vi "Lab Panel V5.29.vi"() -> ()   [LabVIEW 2013] (continued)
                        n3233 = local read "LAB03 TEMP"() -> (w5903:T12)
                        n3234 = call "sub vi - temperature delay v4.vi"("2-run"=w5884, "1-run"=w5885, "temp values IN"=w5902, "temp signals"=w5903) -> ("T2-N"=w5897:dbl, "T2-L"=w5898:dbl, "T1-N"=w5899:dbl, "T1-L"=w5900:dbl, "temp values OUT"=w5901:T44)  [unwired: 3 in]
                        n3235 = Unbundle By Name(w5912) -> ("1 (TL) cal"=w5907:dbl, "1 (TN) cal"=w5906:dbl, "2 (TL) cal"=w5905:dbl, "2 (TN) cal"=w5904:dbl)  [unwired: 6 out]
                        n3236 = local write "TEMP LA03"(w5901) -> ()
                        n3237 = Multiply(x=w5900, y=w5907) -> (x*y=w5893:dbl)
                        n3238 = Multiply(x=w5899, y=w5906) -> (x*y=w5892:dbl)
                        n3239 = Multiply(x=w5898, y=w5905) -> (x*y=w5889:dbl)
                        n3240 = Multiply(x=w5897, y=w5904) -> (x*y=w5888:dbl)
                        n3241 = case shown="True" w5884 {
                          tunnel: w5889 -> [w5914 w5919]
                          tunnel: w5894 -> [_ w5917]
                          tunnel: [w5914 w5918] -> w5887
                          tunnel: w5888 -> [w5913 w5916]
                          tunnel: [w5913 w5915] -> w5886
                          frame False {
                          }
                          frame True {
                            n3242 = Multiply(x=w5917, y=w5916) -> (x*y=w5915:dbl)
                            n3243 = Multiply(x=w5917, y=w5919) -> (x*y=w5918:dbl)
                          }
                        }
                        n3244 = case shown="True" w5885 {
                          tunnel: w5893 -> [w5921 w5926]
                          tunnel: w5894 -> [_ w5924]
                          tunnel: [w5921 w5925] -> w5891
                          tunnel: w5892 -> [w5920 w5923]
                          tunnel: [w5920 w5922] -> w5890
                          frame False {
                          }
                          frame True {
                            n3245 = Multiply(x=w5924, y=w5923) -> (x*y=w5922:dbl)
                            n3246 = Multiply(x=w5924, y=w5926) -> (x*y=w5925:dbl)
                          }
                        }
                        n3247 = local read "SIG LAB03-2"() -> (w5909:T2)
                        n3248 = local read "SIG LAB03-1"() -> (w5911:T2)
                        n3249 = Bundle By Name(cluster=w5911, "Tmp Live"=w5891, "Tmp Neut"=w5890) -> (w5910:T2)
                        n3250 = Bundle By Name(cluster=w5909, "Tmp Live"=w5887, "Tmp Neut"=w5886) -> (w5908:T2)
                        n3251 = local write "SIG LAB03-1"(w5910) -> ()
                        n3252 = local write "SIG LAB03-2"(w5908) -> ()
                      }
                      frame #4 {
                        n3253 = case shown="False" w5941 {
                          tunnel: [w5972 w5973] -> w5957
                          tunnel: w5940 -> [_ w5973]
                          frame False {
                            n3254 = local read "CAL LAB04"() -> (w5972:T14)
                          }
                          frame True {
                          }
                        }
                        n3255 = local read "LAB04 TEMP"() -> (w5947:T12)
                        n3256 = local read "TEMP LA04"() -> (w5948:T9)
                        n3257 = call "sub vi - temperature delay v4.vi"("2-run"=w5929, "1-run"=w5930, "temp values IN"=w5948, "temp signals"=w5947) -> ("T2-N"=w5942:dbl, "T2-L"=w5943:dbl, "T1-N"=w5944:dbl, "T1-L"=w5945:dbl, "temp values OUT"=w5946:T44)  [unwired: 3 in]
                        n3258 = Unbundle By Name(w5957) -> ("1 (TL) cal"=w5952:dbl, "1 (TN) cal"=w5951:dbl, "2 (TL) cal"=w5950:dbl, "2 (TN) cal"=w5949:dbl)  [unwired: 6 out]
                        n3259 = local write "TEMP LA04"(w5946) -> ()
                        n3260 = Multiply(x=w5945, y=w5952) -> (x*y=w5938:dbl)
                        n3261 = Multiply(x=w5944, y=w5951) -> (x*y=w5937:dbl)
                        n3262 = Multiply(x=w5943, y=w5950) -> (x*y=w5934:dbl)
                        n3263 = Multiply(x=w5942, y=w5949) -> (x*y=w5933:dbl)
                        n3264 = case shown="True" w5929 {
                          tunnel: w5934 -> [w5959 w5964]
                          tunnel: w5939 -> [_ w5962]
                          tunnel: [w5959 w5963] -> w5932
                          tunnel: w5933 -> [w5958 w5961]
                          tunnel: [w5958 w5960] -> w5931
                          frame False {
                          }
                          frame True {
                            n3265 = Multiply(x=w5962, y=w5961) -> (x*y=w5960:dbl)
                            n3266 = Multiply(x=w5962, y=w5964) -> (x*y=w5963:dbl)
                          }
                        }
                        n3267 = case shown="True" w5930 {
                          tunnel: w5938 -> [w5966 w5971]
                          tunnel: w5939 -> [_ w5969]
                          tunnel: [w5966 w5970] -> w5936
                          tunnel: w5937 -> [w5965 w5968]
                          tunnel: [w5965 w5967] -> w5935
                          frame False {
                          }
                          frame True {
                            n3268 = Multiply(x=w5969, y=w5968) -> (x*y=w5967:dbl)
                            n3269 = Multiply(x=w5969, y=w5971) -> (x*y=w5970:dbl)
                          }
                        }
                        n3270 = local read "SIG LAB04-2"() -> (w5954:T2)
                        n3271 = local read "SIG LAB04-1"() -> (w5956:T2)
                        n3272 = Bundle By Name(cluster=w5956, "Tmp Live"=w5936, "Tmp Neut"=w5935) -> (w5955:T2)
                        n3273 = Bundle By Name(cluster=w5954, "Tmp Live"=w5932, "Tmp Neut"=w5931) -> (w5953:T2)
                        n3274 = local write "SIG LAB04-1"(w5955) -> ()
                        n3275 = local write "SIG LAB04-2"(w5953) -> ()
                      }
                      frame #5 {
                        n3276 = case shown="False" w5986 {
                          tunnel: [w6017 w6018] -> w6002
                          tunnel: w5985 -> [_ w6018]
                          frame False {
                            n3277 = local read "CAL LAB05"() -> (w6017:T14)
                          }
                          frame True {
                          }
                        }
                        n3278 = local read "LAB05 TEMP"() -> (w5992:T12)
                        n3279 = local read "TEMP LA05"() -> (w5993:T9)
                        n3280 = call "sub vi - temperature delay v4.vi"("2-run"=w5974, "1-run"=w5975, "temp values IN"=w5993, "temp signals"=w5992) -> ("T2-N"=w5988:dbl, "T2-L"=w5989:dbl, "T1-N"=w5990:dbl, "T1-L"=w5991:dbl, "temp values OUT"=w5987:T44)  [unwired: 3 in]
                        n3281 = local write "TEMP LA05"(w5987) -> ()
                        n3282 = Unbundle By Name(w6002) -> ("1 (TL) cal"=w5994:dbl, "1 (TN) cal"=w5997:dbl, "2 (TL) cal"=w5996:dbl, "2 (TN) cal"=w5995:dbl)  [unwired: 6 out]
                        n3283 = Multiply(x=w5991, y=w5994) -> (x*y=w5983:dbl)
                        n3284 = Multiply(x=w5990, y=w5997) -> (x*y=w5982:dbl)
                        n3285 = Multiply(x=w5989, y=w5996) -> (x*y=w5979:dbl)
                        n3286 = Multiply(x=w5988, y=w5995) -> (x*y=w5978:dbl)
                        n3287 = case shown="True" w5974 {
                          tunnel: w5979 -> [w6004 w6009]
                          tunnel: w5984 -> [_ w6007]
                          tunnel: [w6004 w6008] -> w5977
                          tunnel: w5978 -> [w6003 w6006]
                          tunnel: [w6003 w6005] -> w5976
                          frame False {
                          }
                          frame True {
                            n3288 = Multiply(x=w6007, y=w6006) -> (x*y=w6005:dbl)
                            n3289 = Multiply(x=w6007, y=w6009) -> (x*y=w6008:dbl)
                          }
                        }
                        n3290 = case shown="True" w5975 {
                          tunnel: w5983 -> [w6011 w6016]
                          tunnel: w5984 -> [_ w6014]
                          tunnel: [w6011 w6015] -> w5981
                          tunnel: w5982 -> [w6010 w6013]
                          tunnel: [w6010 w6012] -> w5980
                          frame False {
                          }
                          frame True {
                            n3291 = Multiply(x=w6014, y=w6013) -> (x*y=w6012:dbl)
                            n3292 = Multiply(x=w6014, y=w6016) -> (x*y=w6015:dbl)
                          }
                        }
                        n3293 = local read "SIG LAB05-1"() -> (w6001:T2)
                        n3294 = Bundle By Name(cluster=w6001, "Tmp Live"=w5981, "Tmp Neut"=w5980) -> (w6000:T2)
                        n3295 = local read "SIG LAB05-2"() -> (w5999:T2)
                        n3296 = Bundle By Name(cluster=w5999, "Tmp Live"=w5977, "Tmp Neut"=w5976) -> (w5998:T2)
                        n3297 = local write "SIG LAB05-1"(w6000) -> ()
                        n3298 = local write "SIG LAB05-2"(w5998) -> ()
                      }
                      frame #6 {
                        w6119 = 150.0
                        # "check for thermocouple error, output >150 deg??"
                        n3299 = local read "SIG LAB01-2"() -> (w6128:T2)
                        n3300 = local read "SIG LAB04-1"() -> (w6122:T2)
                        n3301 = local read "SIG LAB04-2"() -> (w6123:T2)
                        n3302 = local read "SIG LAB01-1"() -> (w6129:T2)
                        n3303 = Unbundle(w6123) -> ("Tmp Live"=w6033:dbl, "Tmp Neut"=w6032:dbl)  [unwired: 3 out]
                        n3304 = Unbundle(w6128) -> ("Tmp Live"=w6054:dbl, "Tmp Neut"=w6052:dbl)  [unwired: 3 out]
                        n3305 = Unbundle(w6122) -> ("Tmp Live"=w6034:dbl, "Tmp Neut"=w6027:dbl)  [unwired: 3 out]
                        n3306 = Unbundle(w6129) -> ("Tmp Live"=w6057:dbl, "Tmp Neut"=w6055:dbl)  [unwired: 3 out]
                        n3307 = Absolute Value(x=w6034) -> (abs(x)=w6028:dbl)
                        n3308 = Absolute Value(x=w6027) -> (abs(x)=w6029:dbl)
                        n3309 = Absolute Value(x=w6033) -> (abs(x)=w6031:dbl)
                        n3310 = Absolute Value(x=w6032) -> (abs(x)=w6030:dbl)
                        n3311 = Absolute Value(x=w6054) -> (abs(x)=w6053:dbl)
                        n3312 = Absolute Value(x=w6052) -> (abs(x)=w6051:dbl)
                        n3313 = Absolute Value(x=w6055) -> (abs(x)=w6056:dbl)
                        n3314 = Absolute Value(x=w6057) -> (abs(x)=w6058:dbl)
                        n3315 = Greater?(x=w6030, y=w6119) -> (0:w6095:bool)
                        "LA04-2 (TN)" <- w6095
                        n3316 = Greater?(x=w6051, y=w6119) -> (0:w6107:bool)
                        "LA01-2 (TN)" <- w6107
                        n3317 = Greater?(x=w6031, y=w6119) -> (0:w6096:bool)
                        "LA04-2 (TL)" <- w6096
                        n3318 = Greater?(x=w6053, y=w6119) -> (0:w6108:bool)
                        "LA01-2 (TL)" <- w6108
                        n3319 = Greater?(x=w6029, y=w6119) -> (0:w6097:bool)
                        "LA04-1 (TN)" <- w6097
                        n3320 = Greater?(x=w6056, y=w6119) -> (0:w6118:bool)
                        "LA01-1 (TN)" <- w6118
                        n3321 = Greater?(x=w6028, y=w6119) -> (0:w6098:bool)
                        "LA04-1 (TL)" <- w6098
                        n3322 = Greater?(x=w6058, y=w6119) -> (0:w6117:bool)
                        "LA01-1 (TL)" <- w6117
                        n3323 = Or(x=w6118, y=w6117) -> (x .or. y?=w6116:bool)
                        n3324 = Or(x=w6095, y=w6096) -> (x .or. y?=w6106:bool)
                        n3325 = Or(x=w6108, y=w6107) -> (x .or. y?=w6112:bool)
                        n3326 = Or(x=w6097, y=w6098) -> (x .or. y?=w6102:bool)
                        n3327 = Select(t=u32 16711680, s=w6116, f=u32 13816530) -> (s? t:f=w6113:u32)
                        n3328 = Select(t=u32 16711680, s=w6106, f=u32 13816530) -> (s? t:f=w6103:u32)
                        n3329 = Select(t=u32 16711680, s=w6112, f=u32 13816530) -> (s? t:f=w6109:u32)
                        n3330 = Select(t=u32 16711680, s=w6102, f=u32 13816530) -> (s? t:f=w6099:u32)
                        n3331 = property on="SIG LAB01-1" class="Clust (strict)"("Color"=w6113) -> ()  [unwired: 2 in, 2 out]
                        n3332 = property on="SIG LAB01-2" class="Clust (strict)"("Color"=w6109) -> ()  [unwired: 2 in, 2 out]
                        n3333 = property on="SIG LAB04-2" class="Clust (strict)"("Color"=w6103) -> ()  [unwired: 2 in, 2 out]
                        n3334 = property on="SIG LAB04-1" class="Clust (strict)"("Color"=w6099) -> ()  [unwired: 2 in, 2 out]
                        n3335 = local read "SIG LAB02-1"() -> (w6126:T2)
                        n3336 = local read "SIG LAB02-2"() -> (w6127:T2)
                        n3337 = local read "SIG LAB05-2"() -> (w6120:T2)
                        n3338 = local read "SIG LAB05-1"() -> (w6121:T2)
                        n3339 = Unbundle(w6127) -> ("Tmp Live"=w6046:dbl, "Tmp Neut"=w6044:dbl)  [unwired: 3 out]
                        n3340 = Unbundle(w6126) -> ("Tmp Live"=w6050:dbl, "Tmp Neut"=w6049:dbl)  [unwired: 3 out]
                        n3341 = Unbundle(w6120) -> ("Tmp Live"=w6022:dbl, "Tmp Neut"=w6020:dbl)  [unwired: 3 out]
                        n3342 = Unbundle(w6121) -> ("Tmp Live"=w6026:dbl, "Tmp Neut"=w6024:dbl)  [unwired: 3 out]
                        n3343 = Absolute Value(x=w6046) -> (abs(x)=w6045:dbl)
                        n3344 = Absolute Value(x=w6044) -> (abs(x)=w6043:dbl)
                        n3345 = Absolute Value(x=w6049) -> (abs(x)=w6047:dbl)
                        n3346 = Absolute Value(x=w6050) -> (abs(x)=w6048:dbl)
                        n3347 = Absolute Value(x=w6022) -> (abs(x)=w6021:dbl)
                        n3348 = Absolute Value(x=w6020) -> (abs(x)=w6019:dbl)
                        n3349 = Absolute Value(x=w6026) -> (abs(x)=w6025:dbl)
                        n3350 = Absolute Value(x=w6024) -> (abs(x)=w6023:dbl)
                        n3351 = Greater?(x=w6043, y=w6119) -> (0:w6071:bool)
                        "LA02-2 (TN)" <- w6071
                        n3352 = Greater?(x=w6045, y=w6119) -> (0:w6072:bool)
                        "LA02-2 (TL)" <- w6072
                        n3353 = Greater?(x=w6047, y=w6119) -> (0:w6074:bool)
                        "LA02-1 (TN)" <- w6074
                        n3354 = Greater?(x=w6048, y=w6119) -> (0:w6073:bool)
                        "LA02-1 (TL)" <- w6073
                        n3355 = Greater?(x=w6019, y=w6119) -> (0:w6083:bool)
                        "LA05-2 (TN)" <- w6083
                        n3356 = Greater?(x=w6021, y=w6119) -> (0:w6084:bool)
                        "LA05-2 (TL)" <- w6084
                        n3357 = Greater?(x=w6023, y=w6119) -> (0:w6085:bool)
                        "LA05-1 (TN)" <- w6085
                        n3358 = Greater?(x=w6025, y=w6119) -> (0:w6086:bool)
                        "LA05-1 (TL)" <- w6086
                        n3359 = Or(x=w6074, y=w6073) -> (x .or. y?=w6082:bool)
                        n3360 = Or(x=w6072, y=w6071) -> (x .or. y?=w6078:bool)
                        n3361 = Or(x=w6086, y=w6085) -> (x .or. y?=w6094:bool)
                        n3362 = Or(x=w6084, y=w6083) -> (x .or. y?=w6090:bool)
                        n3363 = Select(t=u32 16711680, s=w6082, f=u32 13816530) -> (s? t:f=w6079:u32)
                        n3364 = Select(t=u32 16711680, s=w6078, f=u32 13816530) -> (s? t:f=w6075:u32)
                        n3365 = Select(t=u32 16711680, s=w6094, f=u32 13816530) -> (s? t:f=w6091:u32)
                        n3366 = Select(t=u32 16711680, s=w6090, f=u32 13816530) -> (s? t:f=w6087:u32)
                        n3367 = local read "SIG LAB03-1"() -> (w6124:T2)
                        n3368 = property on="SIG LAB02-1" class="Clust (strict)"("Color"=w6079) -> ()  [unwired: 2 in, 2 out]
                        n3369 = property on="SIG LAB02-2" class="Clust (strict)"("Color"=w6075) -> ()  [unwired: 2 in, 2 out]
                        n3370 = local read "SIG LAB03-2"() -> (w6125:T2)
                        n3371 = property on="SIG LAB05-1" class="Clust (strict)"("Color"=w6091) -> ()  [unwired: 2 in, 2 out]
                        n3372 = property on="SIG LAB05-2" class="Clust (strict)"("Color"=w6087) -> ()  [unwired: 2 in, 2 out]
                        n3373 = Unbundle(w6125) -> ("Tmp Live"=w6038:dbl, "Tmp Neut"=w6036:dbl)  [unwired: 3 out]
                        n3374 = Unbundle(w6124) -> ("Tmp Live"=w6042:dbl, "Tmp Neut"=w6040:dbl)  [unwired: 3 out]
                        n3375 = Absolute Value(x=w6038) -> (abs(x)=w6037:dbl)
                        n3376 = Absolute Value(x=w6036) -> (abs(x)=w6035:dbl)
                        n3377 = Absolute Value(x=w6042) -> (abs(x)=w6041:dbl)
                        n3378 = Absolute Value(x=w6040) -> (abs(x)=w6039:dbl)
                        n3379 = Greater?(x=w6035, y=w6119) -> (0:w6059:bool)
                        "LA03-2 (TN)" <- w6059
                        n3380 = Greater?(x=w6037, y=w6119) -> (0:w6060:bool)
                        "LA03-2 (TL)" <- w6060
                        n3381 = Greater?(x=w6039, y=w6119) -> (0:w6062:bool)
                        "LA03-1 (TN)" <- w6062
                        n3382 = Greater?(x=w6041, y=w6119) -> (0:w6061:bool)
                        "LA03-1 (TL)" <- w6061
                        n3383 = Or(x=w6062, y=w6061) -> (x .or. y?=w6070:bool)
                        n3384 = Or(x=w6060, y=w6059) -> (x .or. y?=w6066:bool)
                        n3385 = Select(t=u32 16711680, s=w6070, f=u32 13816530) -> (s? t:f=w6067:u32)
                        n3386 = Select(t=u32 16711680, s=w6066, f=u32 13816530) -> (s? t:f=w6063:u32)
                        n3387 = property on="SIG LAB03-1" class="Clust (strict)"("Color"=w6067) -> ()  [unwired: 2 in, 2 out]
                        n3388 = property on="SIG LAB03-2" class="Clust (strict)"("Color"=w6063) -> ()  [unwired: 2 in, 2 out]
                      }
                    }
                  }
                }
              }
            }
          }
          frame #22 {
            # "SAVE ON AMPS VALUES FOR REPORT FILE"
            # "write data to display panel"
            n3389 = global write "Global display 1.vi" "TEST 5-2"(w6165) -> ()
            n3390 = global write "Global display 1.vi" "TEST 4-2"(w6167) -> ()
            n3391 = global write "Global display 1.vi" "TEST 1-2"(w6173) -> ()
            n3392 = global write "Global display 1.vi" "TEST 3-1"(w6170) -> ()
            n3393 = global write "Global display 1.vi" "TEST 5-1"(w6166) -> ()
            n3394 = global write "Global display 1.vi" "TEST 1-1"(w6174) -> ()
            n3395 = global write "Global display 1.vi" "TEST 3-2"(w6169) -> ()
            n3396 = global write "Global display 1.vi" "TEST 4-1"(w6168) -> ()
            n3397 = global write "Global display 1.vi" "TEST 2-2"(w6171) -> ()
            n3398 = global write "Global display 1.vi" "TEST 2-1"(w6172) -> ()
            n3399 = global read "Global display 3.vi" "log 1-1"() -> (→"LOG LAB01-1":string)
            n3400 = global read "Global display 3.vi" "log 3-1"() -> (→"LOG LAB03-1":string)
            n3401 = global read "Global display 3.vi" "log 1-2"() -> (→"LOG LAB01-2":string)
            n3402 = property on="Tab Control 2" class="TabCtl (strict)"() -> ("Pages"=w6164:refnum<vi>[])  [unwired: 2 in, 2 out]
            n3403 = global read "Global display 3.vi" "log 2-1"() -> (→"LOG LAB02-1":string)
            n3404 = global read "Global display 3.vi" "log 2-2"() -> (→"LOG LAB02-2":string)
            n3405 = global read "Global display 3.vi" "log 4-2"() -> (→"LOG LAB04-2":string)
            n3406 = global read "Global display 3.vi" "log 5-2"() -> (→"LOG LAB05-2":string)
            n3407 = global read "Global display 3.vi" "log 5-1"() -> (→"LOG LAB05-1":string)
            n3408 = global read "Global display 3.vi" "log 4-1"() -> (→"LOG LAB04-1":string)
            n3409 = global read "Global display 3.vi" "log 3-2"() -> (→"LOG LAB03-2":string)
            n3410 = Index Array(array=w6164, index=8) -> (element=w6162:refnum<vi>)
            n3411 = property class="Page"(reference=w6162) -> ("PageVis"=w6161:bool)  [unwired: 1 in, 2 out]
            n3412 = global write "Global display 3.vi" "admin"(w6161) -> ()
            n3413 = local read "O/I  LAB05-2"() -> (w6215:bool)
            n3414 = local read "O/I  LAB05-1"() -> (w6216:bool)
            n3415 = local read "O/I  LAB03-2"() -> (w6219:bool)
            n3416 = local read "O/I  LAB04-2"() -> (w6217:bool)
            n3417 = local read "O/I  LAB04-1"() -> (w6218:bool)
            n3418 = local read "O/I  LAB03-1"() -> (w6220:bool)
            n3419 = local read "O/I  LAB01-2"() -> (w6223:bool)
            n3420 = local read "O/I  LAB01-1"() -> (w6224:bool)
            n3421 = local read "O/I  LAB02-1"() -> (w6222:bool)
            n3422 = local read "O/I  LAB02-2"() -> (w6221:bool)
            n3423 = global write "Global display 1.vi" "5-2 O/F"(w6215) -> ()
            n3424 = global write "Global display 1.vi" "5-1 O/F"(w6216) -> ()
            n3425 = global write "Global display 1.vi" "4-1 O/F"(w6218) -> ()
            n3426 = global write "Global display 1.vi" "4-2 O/F"(w6217) -> ()
            n3427 = global write "Global display 1.vi" "3-2 O/F"(w6219) -> ()
            n3428 = global write "Global display 1.vi" "3-1 O/F"(w6220) -> ()
            n3429 = global write "Global display 1.vi" "2-2 O/F"(w6221) -> ()
            n3430 = global write "Global display 1.vi" "2-1 O/F"(w6222) -> ()
            n3431 = global write "Global display 1.vi" "1-2 O/F"(w6223) -> ()
            n3432 = global write "Global display 1.vi" "1-1 O/F"(w6224) -> ()
            n3433 = local read "TEMP START LAB02-2"() -> (w6147:cluster{"TL":dbl, "TN":dbl})
            n3434 = local read "run lab05-2"() -> (w6205:bool)
            n3435 = local read "TEMP START LAB01-2"() -> (w6149:cluster{"TL":dbl, "TN":dbl})
            n3436 = local read "TEMP START LAB02-1"() -> (w6148:cluster{"TL":dbl, "TN":dbl})
            n3437 = local read "TEMP START LAB04-1"() -> (w6144:cluster{"TL":dbl, "TN":dbl})
            n3438 = local read "TEMP START LAB04-2"() -> (w6143:cluster{"TL":dbl, "TN":dbl})
            n3439 = local read "run lab04-1"() -> (w6208:bool)
            n3440 = local read "run lab04-2"() -> (w6207:bool)
            n3441 = local read "run lab05-1"() -> (w6206:bool)
            n3442 = local read "TEMP START LAB01-1"() -> (w6150:cluster{"TL":dbl, "TN":dbl})
            n3443 = local read "TEMP START LAB05-2"() -> (w6141:cluster{"TL":dbl, "TN":dbl})
            n3444 = local read "TEMP START LAB05-1"() -> (w6142:cluster{"TL":dbl, "TN":dbl})
            n3445 = local read "run lab03-2"() -> (w6209:bool)
            n3446 = local read "TEMP START LAB03-2"() -> (w6145:cluster{"TL":dbl, "TN":dbl})
            n3447 = local read "TEMP START LAB03-1"() -> (w6146:cluster{"TL":dbl, "TN":dbl})
            n3448 = local read "run lab02-1"() -> (w6212:bool)
            n3449 = local read "run lab03-1"() -> (w6210:bool)
            n3450 = local read "run lab01-2"() -> (w6213:bool)
            n3451 = local read "run lab02-2"() -> (w6211:bool)
            n3452 = local read "run lab01-1"() -> (w6214:bool)
            n3453 = global write "Global display 1.vi" "5-2 R/S"(w6205) -> ()
            n3454 = global write "Global display 1.vi" "5-1 R/S"(w6206) -> ()
            n3455 = global write "Global display 1.vi" "4-2 R/S"(w6207) -> ()
            n3456 = global write "Global display 1.vi" "4-1 R/S"(w6208) -> ()
            n3457 = global write "Global display 1.vi" "3-2 R/S"(w6209) -> ()
            n3458 = global write "Global display 1.vi" "1-2 R/S"(w6213) -> ()
            n3459 = global write "Global display 1.vi" "2-1 R/S"(w6212) -> ()
            n3460 = global write "Global display 1.vi" "3-1 R/S"(w6210) -> ()
            n3461 = global write "Global display 1.vi" "2-2 R/S"(w6211) -> ()
            n3462 = global write "Global display 1.vi" "1-1 R/S"(w6214) -> ()
            n3463 = global write "Global display 3.vi" "TEMP ST 05-2"(w6141) -> ()
            n3464 = global write "Global display 3.vi" "TEMP ST 05-1"(w6142) -> ()
            n3465 = global write "Global display 3.vi" "TEMP ST 03-2"(w6145) -> ()
            n3466 = global write "Global display 3.vi" "TEMP ST 04-2"(w6143) -> ()
            n3467 = global write "Global display 3.vi" "TEMP ST 01-1"(w6150) -> ()
            n3468 = global write "Global display 3.vi" "TEMP ST 01-2"(w6149) -> ()
            n3469 = global write "Global display 3.vi" "TEMP ST 04-1"(w6144) -> ()
            n3470 = global write "Global display 3.vi" "TEMP ST 02-1"(w6148) -> ()
            n3471 = global write "Global display 3.vi" "TEMP ST 02-2"(w6147) -> ()
            n3472 = global write "Global display 3.vi" "TEMP ST 03-1"(w6146) -> ()
            n3473 = local read "DISP LAB04-2"() -> (w6197:T4)
            n3474 = local read "DISP LAB05-1"() -> (w6196:T4)
            n3475 = local read "DISP LAB04-1"() -> (w6198:T4)
            n3476 = local read "DISP LAB05-2"() -> (w6195:T4)
            n3477 = local read "DISP LAB03-2"() -> (w6199:T4)
            n3478 = local read "DISP LAB03-1"() -> (w6200:T4)
            n3479 = local read "DISP LAB01-2"() -> (w6203:T4)
            n3480 = local read "DISP LAB02-1"() -> (w6202:T4)
            n3481 = local read "DISP LAB02-2"() -> (w6201:T4)
            n3482 = local read "DISP LAB01-1"() -> (w6204:T4)
            n3483 = local read "TEMP RISE LAB05-1"() -> (w6132:cluster{"TL":dbl, "TN":dbl})
            n3484 = local read "TEMP RISE LAB05-2"() -> (w6131:cluster{"TL":dbl, "TN":dbl})
            n3485 = local read "TEMP RISE LAB04-2"() -> (w6133:cluster{"TL":dbl, "TN":dbl})
            n3486 = local read "TEMP RISE LAB04-1"() -> (w6134:cluster{"TL":dbl, "TN":dbl})
            n3487 = local read "TEMP RISE LAB03-2"() -> (w6135:cluster{"TL":dbl, "TN":dbl})
            n3488 = local read "TEMP RISE LAB03-1"() -> (w6136:cluster{"TL":dbl, "TN":dbl})
            n3489 = local read "TEMP RISE LAB01-2"() -> (w6139:cluster{"TL":dbl, "TN":dbl})
            n3490 = local read "TEMP RISE LAB02-2"() -> (w6137:cluster{"TL":dbl, "TN":dbl})
            n3491 = local read "TEMP RISE LAB01-1"() -> (w6140:cluster{"TL":dbl, "TN":dbl})
            n3492 = local read "TEMP RISE LAB02-1"() -> (w6138:cluster{"TL":dbl, "TN":dbl})
            n3493 = global write "Global display 2.vi" "DISP LAB05-1"(w6196) -> ()
            n3494 = global write "Global display 2.vi" "DISP LAB05-2"(w6195) -> ()
            n3495 = global write "Global display 2.vi" "DISP LAB04-2"(w6197) -> ()
            n3496 = global write "Global display 2.vi" "DISP LAB04-1"(w6198) -> ()
            n3497 = global write "Global display 2.vi" "DISP LAB02-1"(w6202) -> ()
            n3498 = global write "Global display 2.vi" "DISP LAB02-2"(w6201) -> ()
            n3499 = global write "Global display 2.vi" "DISP LAB03-2"(w6199) -> ()
            n3500 = global write "Global display 2.vi" "DISP LAB01-2"(w6203) -> ()
            n3501 = global write "Global display 2.vi" "DISP LAB01-1"(w6204) -> ()
            n3502 = global write "Global display 2.vi" "DISP LAB03-1"(w6200) -> ()
            n3503 = global write "Global display 3.vi" "TEMP RS 05-2"(w6131) -> ()
            n3504 = global write "Global display 3.vi" "TEMP RS 05-1"(w6132) -> ()
            n3505 = global write "Global display 3.vi" "TEMP RS 03-2"(w6135) -> ()
            n3506 = global write "Global display 3.vi" "TEMP RS 02-1"(w6138) -> ()
            n3507 = global write "Global display 3.vi" "TEMP RS 02-2"(w6137) -> ()
            n3508 = global write "Global display 3.vi" "TEMP RS 04-2"(w6133) -> ()
            n3509 = global write "Global display 3.vi" "TEMP RS 01-2"(w6139) -> ()
            n3510 = global write "Global display 3.vi" "TEMP RS 03-1"(w6136) -> ()
            n3511 = global write "Global display 3.vi" "TEMP RS 04-1"(w6134) -> ()
            n3512 = global write "Global display 3.vi" "TEMP RS 01-1"(w6140) -> ()
            n3513 = local read "SET LAB05-2"() -> (w6185:T5)
            n3514 = local read "SET LAB05-1"() -> (w6186:T5)
            n3515 = local read "SET LAB04-1"() -> (w6188:T5)
            n3516 = local read "SET LAB04-2"() -> (w6187:T5)
            n3517 = local read "SET LAB01-1"() -> (w6194:T5)
            n3518 = local read "SET LAB03-1"() -> (w6190:T5)
            n3519 = local read "SET LAB03-2"() -> (w6189:T5)
            n3520 = local read "SET LAB02-2"() -> (w6191:T5)
            n3521 = local read "SET LAB01-2"() -> (w6193:T5)
            n3522 = local read "SET LAB02-1"() -> (w6192:T5)
            n3523 = global write "Global display 2.vi" "SET LAB05-2"(w6185) -> ()
            n3524 = global write "Global display 2.vi" "SET LAB05-1"(w6186) -> ()
            n3525 = global write "Global display 2.vi" "SET LAB04-1"(w6188) -> ()
            n3526 = global write "Global display 2.vi" "SET LAB01-1"(w6194) -> ()
            n3527 = global write "Global display 2.vi" "SET LAB04-2"(w6187) -> ()
            n3528 = global write "Global display 2.vi" "SET LAB03-2"(w6189) -> ()
            n3529 = global write "Global display 2.vi" "SET LAB02-2"(w6191) -> ()
            n3530 = global write "Global display 2.vi" "SET LAB03-1"(w6190) -> ()
            n3531 = global write "Global display 2.vi" "SET LAB01-2"(w6193) -> ()
            n3532 = global write "Global display 2.vi" "SET LAB02-1"(w6192) -> ()
            n3533 = local read "RESULT LAB01-1"() -> (w6184:bool)
            n3534 = local read "RESULT LAB03-2"() -> (w6179:bool)
            n3535 = local read "RESULT LAB04-1"() -> (w6178:bool)
            n3536 = local read "RESULT LAB04-2"() -> (w6177:bool)
            n3537 = local read "RESULT LAB02-2"() -> (w6181:bool)
            n3538 = local read "RESULT LAB01-2"() -> (w6183:bool)
            n3539 = local read "RESULT LAB02-1"() -> (w6182:bool)
            n3540 = local read "RESULT LAB03-1"() -> (w6180:bool)
            n3541 = local read "RESULT LAB05-1"() -> (w6176:bool)
            n3542 = local read "RESULT LAB05-2"() -> (w6175:bool)
            n3543 = global write "Global display 2.vi" "RESULT LAB05-1"(w6176) -> ()
            n3544 = global write "Global display 2.vi" "RESULT LAB01-2"(w6183) -> ()
            n3545 = global write "Global display 2.vi" "RESULT LAB03-2"(w6179) -> ()
            n3546 = global write "Global display 2.vi" "RESULT LAB04-1"(w6178) -> ()
            n3547 = global write "Global display 2.vi" "RESULT LAB04-2"(w6177) -> ()
            n3548 = global write "Global display 2.vi" "RESULT LAB05-2"(w6175) -> ()
            n3549 = global write "Global display 2.vi" "RESULT LAB03-1"(w6180) -> ()
            n3550 = global write "Global display 2.vi" "RESULT LAB02-1"(w6182) -> ()
            n3551 = global write "Global display 2.vi" "RESULT LAB02-2"(w6181) -> ()
            n3552 = global write "Global display 2.vi" "RESULT LAB01-1"(w6184) -> ()
            n3553 = local read "Amps Fail level"() -> (w6130:dbl)
            n3554 = stacked-sequence {
              tunnel: w6130 -> [w6226 w6231 w6236 w6241 w6246 w6251 w6256 w6261 w6266 w6271]
              frame #0 {
                n3555 = local read "SIG LAB01-1"() -> (w6228:T2)
                n3556 = Unbundle(w6228) -> ("AMPS"=w6227:dbl)  [unwired: 4 out]
                n3557 = Greater?(x=w6227, y=w6226) -> (0:w6225:bool)
                n3558 = case shown="True" w6225 {
                  frame False {
                  }
                  frame True {
                    n3559 = local read "ON L01-1"() -> (w6229:cluster{"amps":dbl, "volts":dbl, "pf":dbl})
                    n3560 = global write "Global display 2.vi" "ON L01-1"(w6229) -> ()
                  }
                }
              }
              frame #1 {
                n3561 = local read "SIG LAB01-2"() -> (w6233:T2)
                n3562 = Unbundle(w6233) -> ("AMPS"=w6232:dbl)  [unwired: 4 out]
                n3563 = Greater?(x=w6232, y=w6231) -> (0:w6230:bool)
                n3564 = case shown="True" w6230 {
                  frame False {
                  }
                  frame True {
                    n3565 = local read "ON L01-2"() -> (w6234:cluster{"amps":dbl, "volts":dbl, "pf":dbl})
                    n3566 = global write "Global display 2.vi" "ON L01-2"(w6234) -> ()
                  }
                }
              }
              frame #2 {
                n3567 = local read "SIG LAB02-1"() -> (w6238:T2)
                n3568 = Unbundle(w6238) -> ("AMPS"=w6237:dbl)  [unwired: 4 out]
                n3569 = Greater?(x=w6237, y=w6236) -> (0:w6235:bool)
                n3570 = case shown="True" w6235 {
                  frame False {
                  }
                  frame True {
                    n3571 = local read "ON L02-1"() -> (w6239:cluster{"amps":dbl, "volts":dbl, "pf":dbl})
                    n3572 = global write "Global display 2.vi" "ON L02-1"(w6239) -> ()
                  }
                }
              }
              frame #3 {
                n3573 = local read "SIG LAB02-2"() -> (w6243:T2)
                n3574 = Unbundle(w6243) -> ("AMPS"=w6242:dbl)  [unwired: 4 out]
                n3575 = Greater?(x=w6242, y=w6241) -> (0:w6240:bool)
                n3576 = case shown="True" w6240 {
                  frame False {
                  }
                  frame True {
                    n3577 = local read "ON L02-2"() -> (w6244:cluster{"amps":dbl, "volts":dbl, "pf":dbl})
                    n3578 = global write "Global display 2.vi" "ON L02-2"(w6244) -> ()
                  }
                }
              }
              frame #4 {
                n3579 = local read "SIG LAB03-1"() -> (w6248:T2)
                n3580 = Unbundle(w6248) -> ("AMPS"=w6247:dbl)  [unwired: 4 out]
                n3581 = Greater?(x=w6247, y=w6246) -> (0:w6245:bool)
                n3582 = case shown="True" w6245 {
                  frame False {
                  }
                  frame True {
                    n3583 = local read "ON L03-1"() -> (w6249:cluster{"amps":dbl, "volts":dbl, "pf":dbl})
                    n3584 = global write "Global display 2.vi" "ON L03-1"(w6249) -> ()
                  }
                }
              }
              frame #5 {
                n3585 = local read "SIG LAB03-2"() -> (w6253:T2)
                n3586 = Unbundle(w6253) -> ("AMPS"=w6252:dbl)  [unwired: 4 out]
                n3587 = Greater?(x=w6252, y=w6251) -> (0:w6250:bool)
                n3588 = case shown="True" w6250 {
                  frame False {
                  }
                  frame True {
                    n3589 = local read "ON L03-2"() -> (w6254:cluster{"amps":dbl, "volts":dbl, "pf":dbl})
                    n3590 = global write "Global display 2.vi" "ON L03-2"(w6254) -> ()
                  }
                }
              }
              frame #6 {
                n3591 = local read "SIG LAB04-1"() -> (w6258:T2)
                n3592 = Unbundle(w6258) -> ("AMPS"=w6257:dbl)  [unwired: 4 out]
                n3593 = Greater?(x=w6257, y=w6256) -> (0:w6255:bool)
                n3594 = case shown="True" w6255 {
                  frame False {
                  }
                  frame True {
                    n3595 = local read "ON L04-1"() -> (w6259:cluster{"amps":dbl, "volts":dbl, "pf":dbl})
                    n3596 = global write "Global display 2.vi" "ON L04-1"(w6259) -> ()
                  }
                }
              }
              frame #7 {
                n3597 = local read "SIG LAB04-2"() -> (w6263:T2)
                n3598 = Unbundle(w6263) -> ("AMPS"=w6262:dbl)  [unwired: 4 out]
                n3599 = Greater?(x=w6262, y=w6261) -> (0:w6260:bool)
                n3600 = case shown="True" w6260 {
                  frame False {
                  }
                  frame True {
                    n3601 = local read "ON L04-2"() -> (w6264:cluster{"amps":dbl, "volts":dbl, "pf":dbl})
                    n3602 = global write "Global display 2.vi" "ON L04-2"(w6264) -> ()
                  }
                }
              }
              frame #8 {
                n3603 = local read "SIG LAB05-1"() -> (w6268:T2)
                n3604 = Unbundle(w6268) -> ("AMPS"=w6267:dbl)  [unwired: 4 out]
                n3605 = Greater?(x=w6267, y=w6266) -> (0:w6265:bool)
                n3606 = case shown="True" w6265 {
                  frame False {
                  }
                  frame True {
                    n3607 = local read "ON L05-1"() -> (w6269:cluster{"amps":dbl, "volts":dbl, "pf":dbl})
                    n3608 = global write "Global display 2.vi" "ON L05-1"(w6269) -> ()
                  }
                }
              }
              frame #9 {
                n3609 = local read "SIG LAB05-2"() -> (w6273:T2)
                n3610 = Unbundle(w6273) -> ("AMPS"=w6272:dbl)  [unwired: 4 out]
                n3611 = Greater?(x=w6272, y=w6271) -> (0:w6270:bool)
                n3612 = case shown="True" w6270 {
                  frame False {
                  }
                  frame True {
                    n3613 = local read "ON L05-2"() -> (w6274:cluster{"amps":dbl, "volts":dbl, "pf":dbl})
                    n3614 = global write "Global display 2.vi" "ON L05-2"(w6274) -> ()
                  }
                }
              }
            }
          }
          frame #23 {
            # "simulate values"
            n3615 = global write "Global display 4.vi" "LAB deg C"("LAB deg C") -> ()
          }
          frame #24 {
            # "end main and display program"
            n3616 = stacked-sequence {
              seq-local: [_ w6281 _] -> [_ _ w6287]
              tunnel: w6277 -> [w6278 _ _]
              tunnel: w6276 -> [_ _ w6285]
              frame #0 {
                n3617 = case shown="True" w6278 {
                  frame False {
                  }
                  frame True {
                    n3618 = One Button Dialog(message="Excessive number of USB \nresets done, re-start program.") -> ()  [unwired: 1 in, 1 out]
                  }
                }
              }
              frame #1 {
                # "check for reset error"
                n3619 = local read "Simulate"() -> (w6280:bool)
                n3620 = case shown="False" w6280 {
                  tunnel: [w6282 FALSE] -> w6281
                  frame False {
                    n3621 = local read "Reset Error"() -> (w6282:bool)
                    n3622 = case shown="True" w6282 {
                      frame False {
                      }
                      frame True {
                        n3623 = One Button Dialog(message="USB ERROR, program will be stopped.\nClose program, close windows, switch panel off\nand re power panel. If error persists seek help.") -> ()  [unwired: 1 in, 1 out]
                      }
                    }
                  }
                  frame True {
                  }
                }
              }
              frame #2 {
                # "end labview session"
                n3624 = case shown="True" w6285 {
                  frame False {
                  }
                  frame True {
                    n3625 = call "sub vi - AI USB4704 (3)  Close Task v2.vi"() -> ()  [unwired: 16 in]
                  }
                }
                n3626 = Or(x=w6287, y="stop all") -> (x .or. y?=w6286:bool)
                n3627 = case shown="True" w6286 {
                  frame False {
                  }
                  frame True {
                    n3628 = stacked-sequence {
                      frame #0 {
                        n3629 = global write "Global display 1.vi" "stop disp"(TRUE) -> ()
                      }
                      frame #1 {
                        n3630 = call "sub vi - AI USB4704 (3)  Close Task v2.vi"() -> ()  [unwired: 16 in]
                      }
                      frame #2 {
                        n3631 = Quit LabVIEW(quit? (T)=TRUE) -> ()
                      }
                    }
                  }
                }
              }
            }
          }
        }
        n3632 = node-c288() -> ()  [unwired: 1 in, 1 out]
        "loops" <- w350
      }
      n3633 = node-c288(w322) -> ()  [unwired: 1 out]
    }
  }
